vi "CoolProp_HAProp_SI_V15.0.vi"(4 "Value2":dbl=1.0, 5 "Value1":dbl=400.0, 6 "Humidity parameter":T1(ring), 7 "Dry bulb temperature of moist air":enum16{"T [K]"}(ring), 8 "error in (no error)":errorcluster, 9 "Output":string="H", 11 "path in":path=path "C:/Program Files (x86)/National Instruments/LabVIEW 2015/user.lib/CoolProp.dll") -> (0 "error out":errorcluster, 2 "error_message":string, 3 "Return Value":dbl=416.75835925510785)   [LabVIEW 2015]
panel:
  in  "Absolute pressure of moist air":enum16{"P [Pa]"}(ring)
  in  "Value3":dbl=1.0
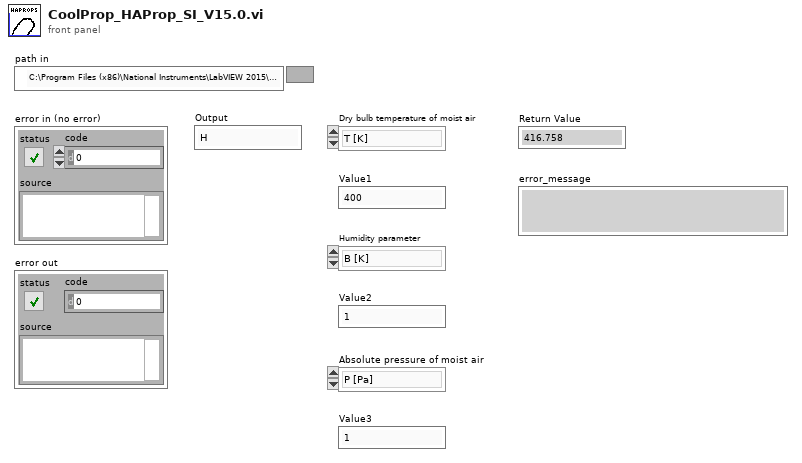
[diagram p1: front panel]
types:
  T1 = enum16{"B [K]", "D [K]", "R [-]", "W [kg wv/kg da]"}
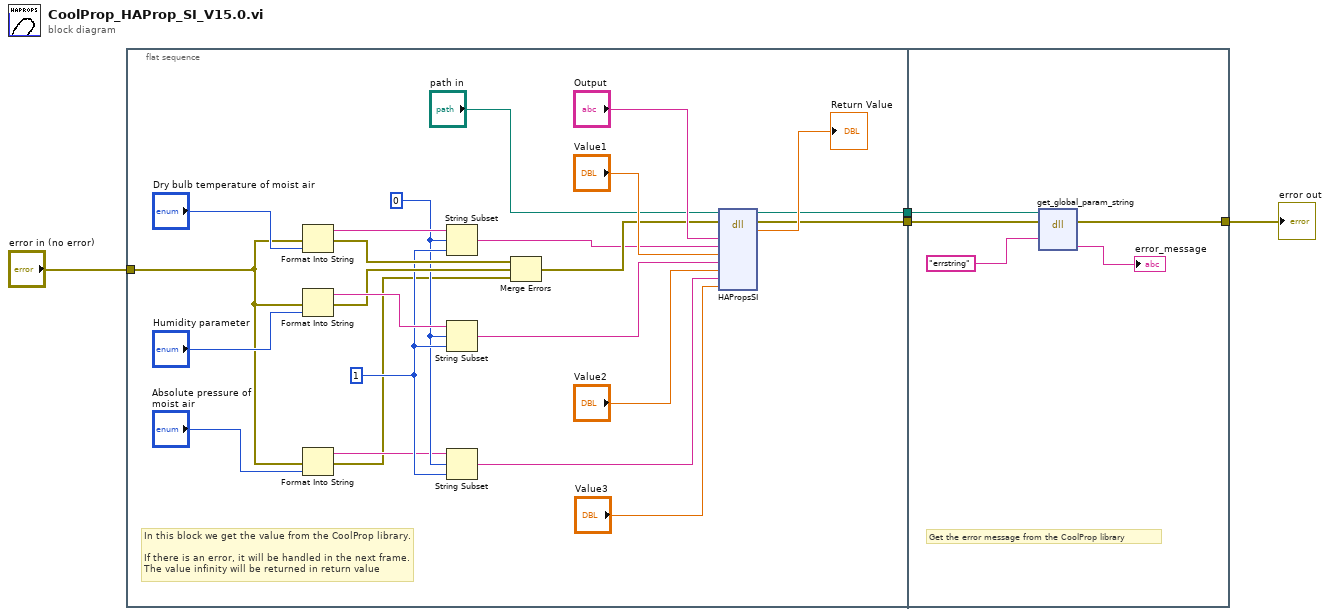
[diagram p0: block diagram]
diagram:
  n1 = flat-sequence {
    tunnel: "error in (no error)" -> [w8]
    tunnel: [w15] -> w3
    tunnel: [w14] -> w1
    tunnel: w3 -> [w31]
    tunnel: [w30] -> w2
    tunnel: w1 -> [w29]
    frame #0 {
      w11 = 1 ("length (rest)")
      w10 = 0 ("offset (0)")
      # "In this block we get the value from the CoolProp library.\n\nIf there is an error, it will be handled in the next frame.\nThe value infinity will be returned in return value"
      n2 = Format Into String(error in=w8, "Dry bulb temperature of moist air") -> (resulting string=w24:string, error out=w22:errorcluster)  [unwired: 2 in]
      n3 = Format Into String(error in=w8, "Humidity parameter") -> (resulting string=w23:string, error out=w21:errorcluster)  [unwired: 2 in]
      n4 = Format Into String(error in=w8, "Absolute pressure of moist air") -> (resulting string=w7:string, error out=w5:errorcluster)  [unwired: 2 in]
      n5 = String Subset(string=w24, offset (0)=w10, length (rest)=w11) -> (substring=w17:string)
      n6 = String Subset(string=w23, offset (0)=w10, length (rest)=w11) -> (substring=w16:string)
      n7 = String Subset(string=w7, offset (0)=w10, length (rest)=w11) -> (substring=w6:string)
      n8 = Merge Errors(w22, w21, w5) -> (w20:errorcluster)
      n9 = dll-call lib="C:/Program Files (x86)/National Instruments/LabVIEW 2015/user.lib/CoolProp.dll" fn="HAPropsSI"(path in="path in", error in=w20, "Output"="Output", "Input1"=w17, "Value1"="Value1", "Input2"=w16, "Value2"="Value2", "Input3"=w6, "Value3"="Value3") -> (path out=w14:path, error out=w15:errorcluster, "OutputValue"=→"Return Value":dbl)  [unwired: 8 in]
    }
    frame #1 {
      # "Get the error message from the CoolProp library"
      n10 = dll-call lib="C:/Program Files (x86)/National Instruments/LabVIEW 2011/user.lib/CoolProp.dll" fn="get_global_param_string"(path in=w29, error in=w31, "param"="errstring") -> (error out=w30:errorcluster, "error_message"=→"error_message":string)  [unwired: 2 in, 3 out]
    }
  }
  "error out" <- w2
